vi "Dashboard Main.vi"() -> ()   [LabVIEW 2013]
uses:
  <vilib>/event_ctls.llb/eventvkey.ctl
  <vilib>/Utility/config.llb/NI_LVConfig.lvlib
  <vilib>/Utility/config.llb/Write Key (I32).vi
  <vilib>/Rock Robotics/WPI/Dashboard/WPI_DashboardLogging Global.vi
  <vilib>/Utility/config.llb/Write Key (String).vi
  2014 Robot Project/Robot Global Data.vi
panel:
  out "Image Message":string="Timeout in Camera Communications"
  in  "Rec Mode":enum32{"Stop", "Record", "Playback"}(radio)
  in  "Dashboard Tab":T1(tab)
  in  "Camera Settings":T2={"Frame Rate"=30, "Compression"=30, "Size"=1} {"Frame Rate" scale=1.0..30.0; "Size" items=["640x480", "320x240", "160x120"]}
  in  "DB Camera Config":bool
  out "fps":dbl format="%#.1g"
  out "Mbps":dbl format="%#.1g"
  out "Mbps 2":bool
  out "LED 1":bool
  in  "Slider 1":dbl(slide) scale=0.0..100.0
  in  "Checkbox 2":bool
  in  "Checkbox 1":bool
  in  "Test Slider":dbl(slide) scale=0.0..100.0 scale format="%#_3g"
  in  "On/Off":bool caption="Solenoid"
  in  "Test Name":u16(ring) items=["Select the test to run...", "Example Test", "-------------------------------", "List of tests is built in robot code.", "Replace with your own automated tests."]
  in  "Test Tree":string(tree)
  in  "Motor":cluster{"Value":dbl, "Enable":bool} {"Value" scale=-1.0..1.0 scale format="%#_3g"}
  out "Progress":T3 {"Test Progress" scale=0.0..100.0}
  in  "Rev/Fwd":cluster{"Forward":bool, "Reverse":bool}
  in  "Test Ring":u16(ring) items=["Auto", "Fixed indoor", "Fixed outdoor 1", "Fixed outdoor 2", "Fixed fluorescent 1", "Fixed fluorescent 2", "Hold current"]
  in  "Listbox":i32(listbox)
  out "Tree":string(tree)
  out "Camera Image":T4(plugin-control)
  in  "Enable":bool
  # "Left"
  # "Front"
  # "Right"
  # "Battery"
  # "Customize by placing controls and indicators here and name to\nmatch Dashboard Variables on robot."
  # "This tab is a great place for autonomous settings and validation.\nCustomize by placing controls and indicators here and name to\nmatch Dashboard Variables on robot."
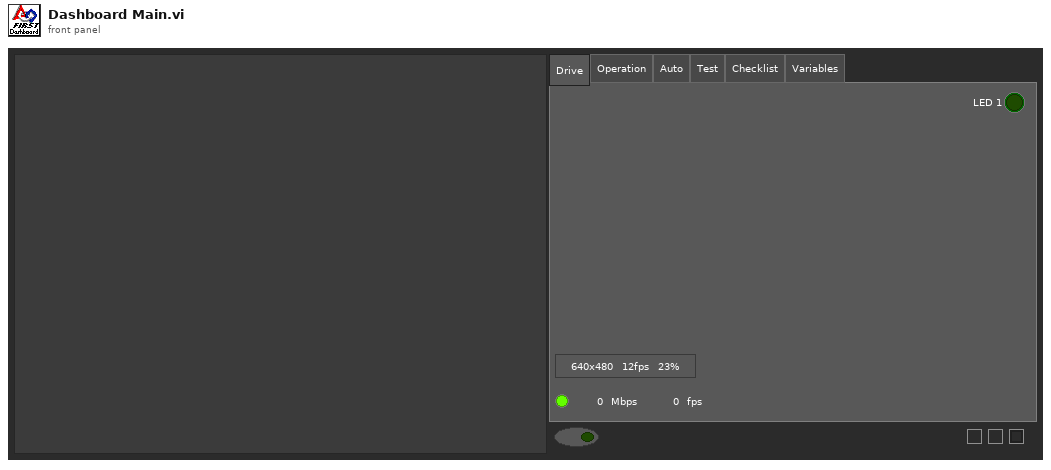
[diagram p1: front panel]
types:
  T1 = enum32{"Drive", "Operation", "Auto", "Test", "Checklist", "Variables"}
  T2 = cluster{"Frame Rate":i32, "Compression":i32, "Size":u16}
  T3 = cluster{"Test Progress":u8, "Test Progress Text":string}
  T4 = typedef "IMAQ Image.ctl" = refnum<image>
  T5 = typedef "Image Type" = u32
  T6 = typedef "NI_LVConfig.lvlib/Config Data RefNum.ctl" = refnum<k1>
  T7 = typedef "eventvkey.ctl" = enum16{"ASCII", "Enter", "Return", "Shift", "Ctrl", "Alt", "Cmd", "Opt", "Caps", "NumLock", "Clear", "Break", "Up", "Down", "Left", "Right", "Insert", "Delete", "Home", "End", "PageUp", "PageDown", "Escape", "Help", "Pause", "ScrollLock", "F1", "F2", "F3", "F4", "F5", "F6", "F7", "F8", "F9", "F10", "F11", "F12", "F13", "F14", "F15", "F16", "F17", "F18", "F19", "F20", "F21", "F22", "F23", "F24", "Play", "VolumeUp", "VolumeDown", "Mute", "Two Byte Char"}
  T8 = cluster{"Image Size":bool, "Image Type":bool, "Pixel Value":bool, "ROI Information":bool, "Zoom Factor":bool}
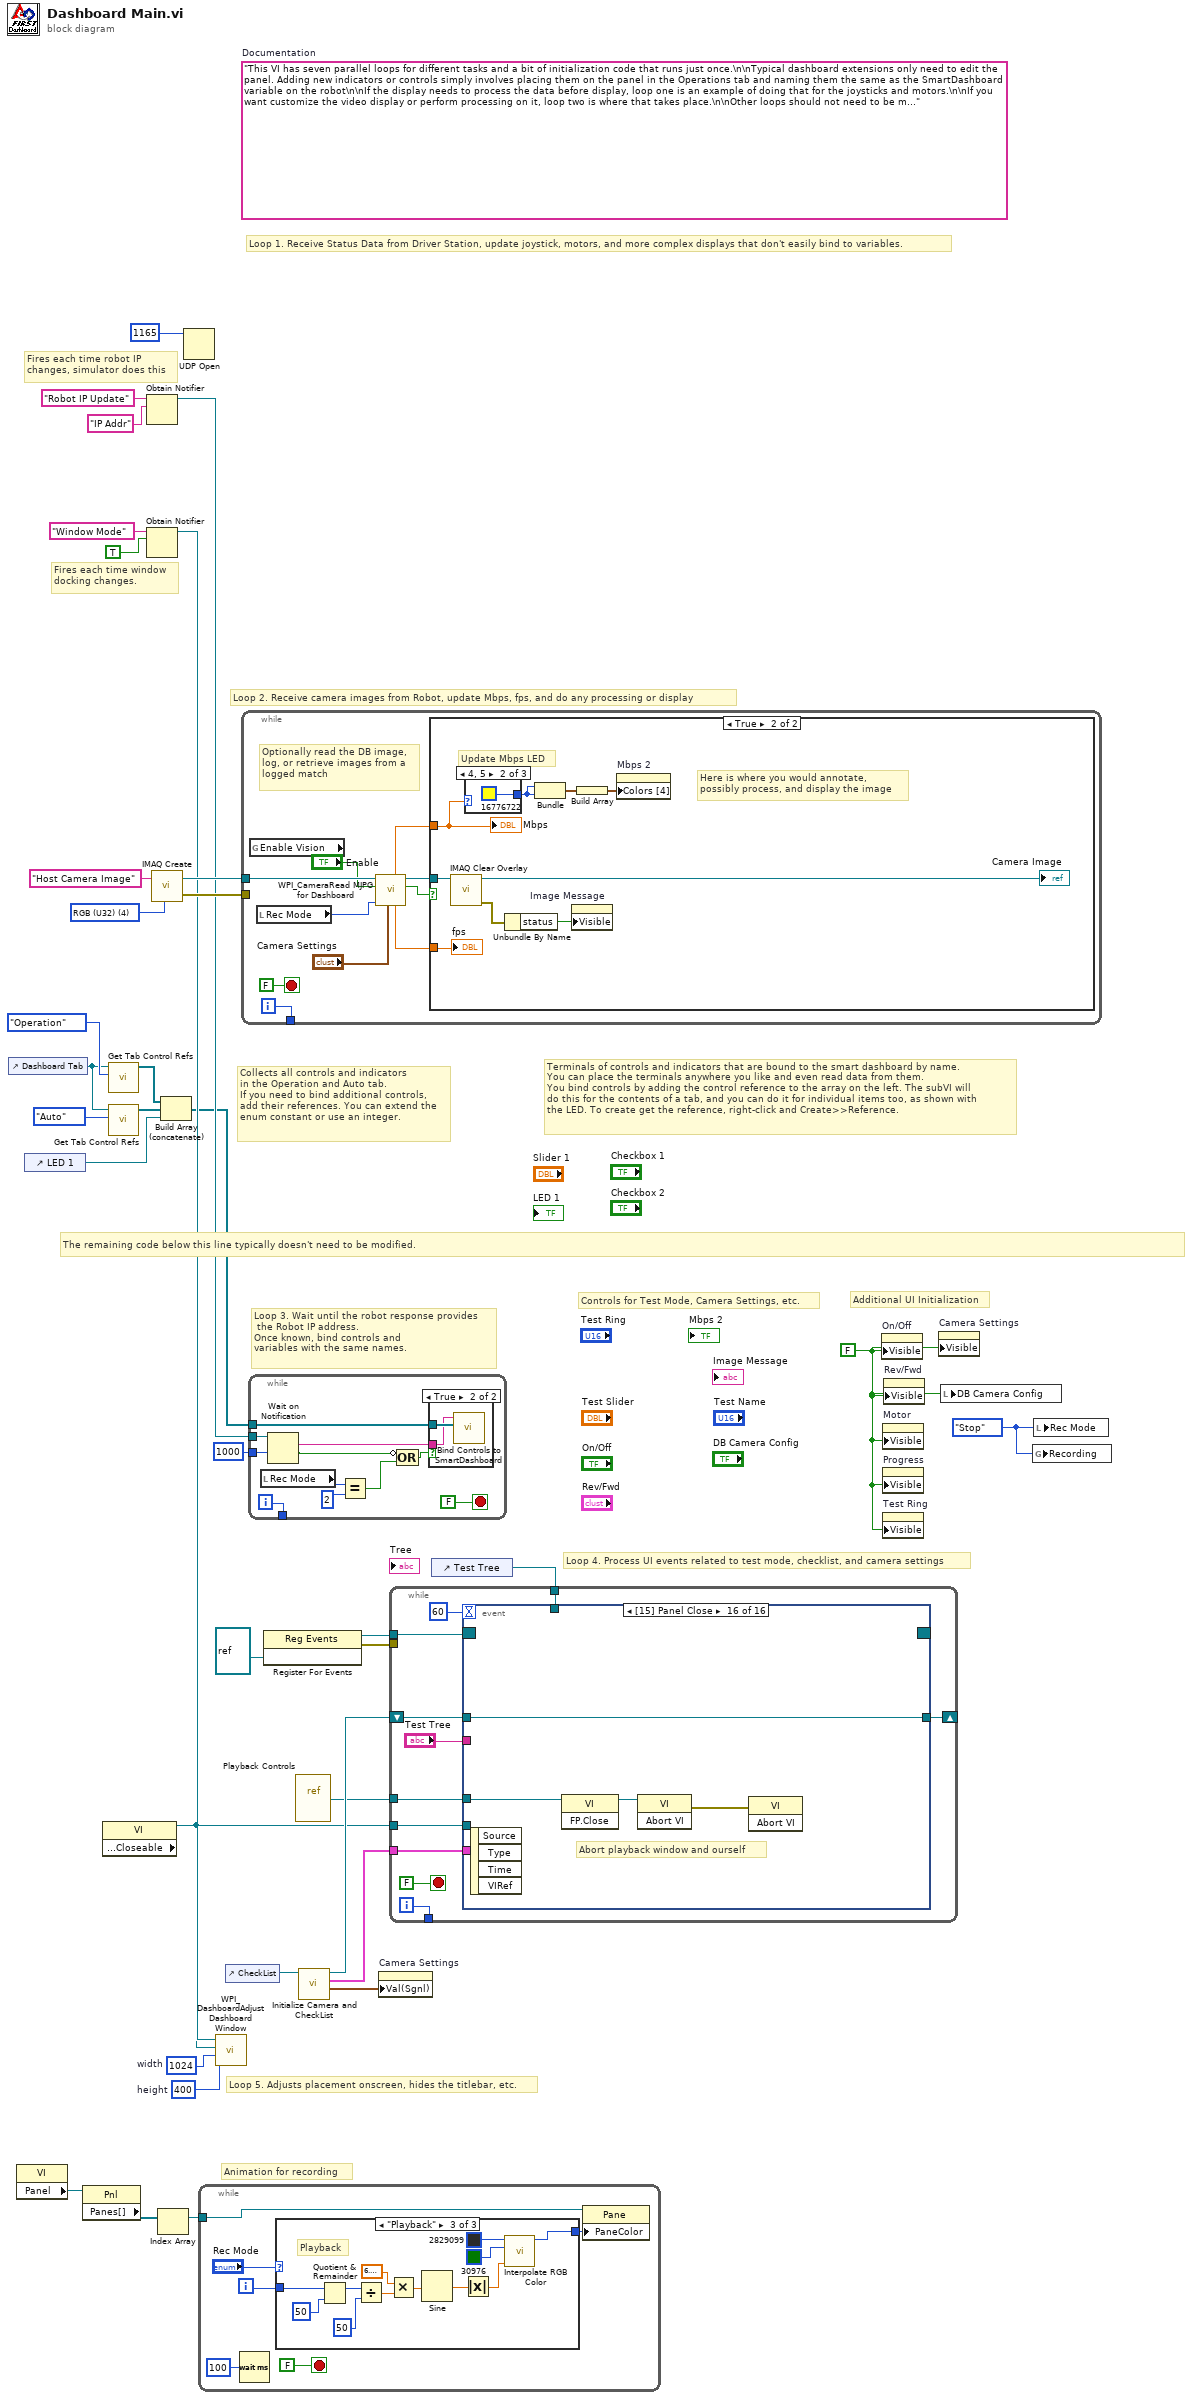
[diagram p0: block diagram]
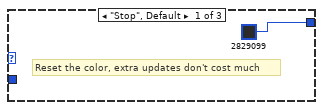
[diagram p2: hidden frame]
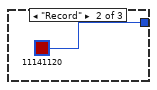
[diagram p3: hidden frame]
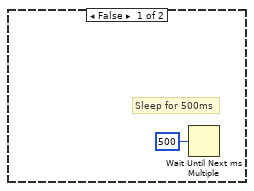
[diagram p5: hidden frame]
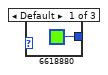
[diagram p6: hidden frame]
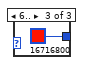
[diagram p7: hidden frame]
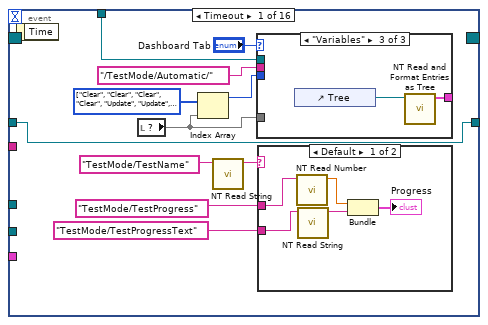
[diagram p8: hidden frame]
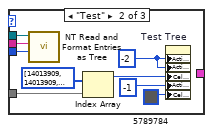
[diagram p10: hidden frame]
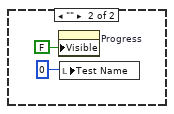
[diagram p11: hidden frame]
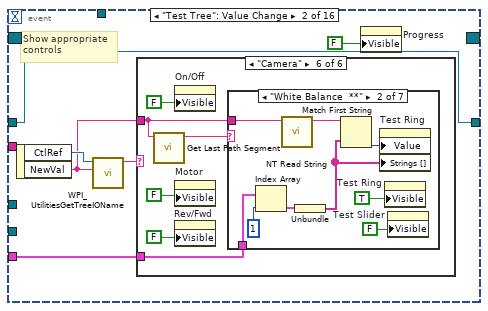
[diagram p12: hidden frame]
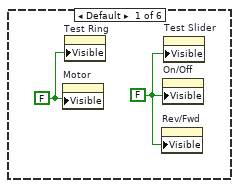
[diagram p13: hidden frame]
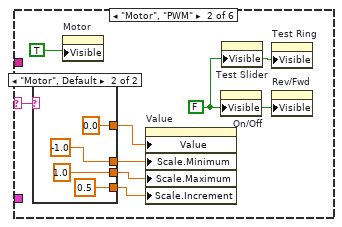
[diagram p14: hidden frame]
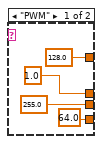
[diagram p15: hidden frame]
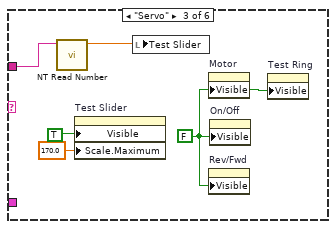
[diagram p16: hidden frame]
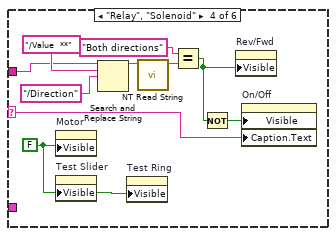
[diagram p17: hidden frame]
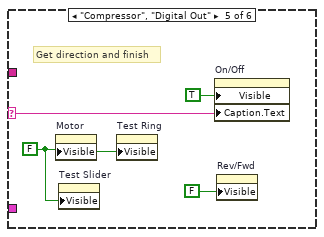
[diagram p18: hidden frame]
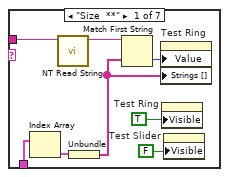
[diagram p19: hidden frame]
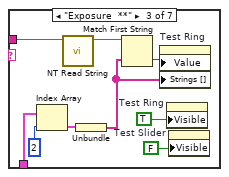
[diagram p20: hidden frame]
diagram:
  w8 = enum32{"Stop", "Record", "Playback"}."Stop" ("Rec Mode")
  w11 = 400  # height
  w12 = 1024  # width
  w25 = FALSE ("Visible")
  (unwired) "This VI has seven parallel loops for different tasks and a bit of initialization code that runs just once.\n\nTypical dashboard extensions only need to edit the panel. Adding new indicators or controls simply involves placing them on the panel in the Operations tab and naming them the same as the SmartDashboard variable on the robot\n\nIf the display needs to process the data before display, loop one is an example of doing that for the joysticks and motors.\n\nIf you want customize the video display or perform processing on it, loop two is where that takes place.\n\nOther loops should not need to be modified. They are pretty standard, and document the task they perform."  # Documentation
  w35 = T5 4 items=["Grayscale (U8)", "Grayscale (I16)", "Grayscale (SGL)", "Complex (CSG)", "RGB (U32)", "HSL (U32)", "RGB (U64)"] ("Image Type")
  # "Controls for Test Mode, Camera Settings, etc."
  # "Additional UI Initialization"
  # "Animation for recording"
  # "Fires each time robot IP\nchanges, simulator does this"
  # "Fires each time window\ndocking changes."
  # "Collects all controls and indicators\nin the Operation and Auto tab.\nIf you need to bind additional controls,\nadd their references. You can extend the\nenum constant or use an integer."
  # "The remaining code below this line typically doesn't need to be modified."
  # "Loop 4. Process UI events related to test mode, checklist, and camera settings"
  # "Terminals of controls and indicators that are bound to the smart dashboard by name.\nYou can place the terminals anywhere you like and even read data from them.\nYou bind controls by adding the control reference to the array on the left. The subVI will\ndo this for the contents of a tab, and you can do it for individual items too, as shown with\nthe LED. To create get the reference, right-click and Create>>Reference."
  # "Loop 3. Wait until the robot response provides\n the Robot IP address.\nOnce known, bind controls and\nvariables with the same names."
  # "Loop 5. Adjusts placement onscreen, hides the titlebar, etc."
  # "Loop 1. Receive Status Data from Driver Station, update joystick, motors, and more complex displays that don't easily bind to variables."
  # "Loop 2. Receive camera images from Robot, update Mbps, fps, and do any processing or display"
  n1 = control-ref of="Dashboard Tab"() -> (w6:refnum<vi>)
  n2 = property class="VI"() -> ("Panel"=w19:refnum<vi>)  [unwired: 2 in, 2 out]
  n3 = control-ref of="LED 1"() -> (w1:refnum<vi>)
  n4 = property class="Pnl"(reference=w19) -> ("Panes[]"=w20:refnum<vi>[])  [unwired: 1 in, 2 out]
  n5 = property class="VI" props=["Front Panel.Closeable"]() -> (reference out=w7:refnum<vi>)  [unwired: 2 in, 2 out]
  n6 = call <vilib>:"Get Tab Control Refs.vi"("Page Index"=T1."Operation" ("Dashboard Tab"), "TabControl in"=w6) -> ("ControlsOnPage"=w4:refnum<vi>[])  [unwired: 9 in]
  n7 = call <vilib>:"Get Tab Control Refs.vi"("Page Index"=T1."Auto" ("Dashboard Tab"), "TabControl in"=w6) -> ("ControlsOnPage"=w5:refnum<vi>[])  [unwired: 9 in]
  n8 = Obtain Notifier(name (unnamed)="Robot IP Update", notification data type="IP Addr" ("name (unnamed)")) -> (notifier out=w29:refnum<notifier>)  [unwired: 2 in, 2 out]
  n9 = Obtain Notifier(name (unnamed)="Window Mode", notification data type=TRUE) -> (notifier out=w10:refnum<notifier>)  [unwired: 2 in, 2 out]
  n10 = call "IMAQ Create"("Image Name"="Host Camera Image", "Image Type"=w35) -> ("New Image"=w33:T4, "error out"=w32:errorcluster)  [unwired: 2 in, 1 out]
  n11 = Index Array(array=w20) -> (element=w18:refnum<vi>)  [unwired: 1 in]
  n12 = Build Array (concatenate)(w4, w5, w1) -> (w3:refnum<vi>[])
  n13 = UDP Open(11:u16 1165 ("port")) -> (port=w36:refnum<k16>)  [unwired: 2 in, 4 out]
  n14 = while {
    tunnel: w18 -> [w39]
    i -> [w42]
    stop <- FALSE stop-if-true
    n15 = Wait (ms)(milliseconds to wait=u32 100) -> ()  [unwired: 1 out]
    n16 = case shown="\"Playback\"" "Rec Mode" {
      tunnel: w42 -> [_ _ w57]
      tunnel: [u32 2829099 ("Base Color") u32 11141120 ("Target Color") w46] -> w38
      frame "Stop", Default {
        # "Reset the color, extra updates don't cost much"
      }
      frame "Record" {
      }
      frame "Playback" {
        # "Playback"
        n17 = Quotient & Remainder(x=w57, y=u32 50 ("milliseconds to wait")) -> (x-y*floor(x/y)=w53:u32)  [unwired: 1 out]
        n18 = Divide(x=w53, y=u32 50 ("milliseconds to wait")) -> (x/y=w50:dbl)
        n19 = Multiply(x=6.283185307179586, y=w50) -> (x*y=w55:dbl)
        n20 = Sine(x=w55) -> (sin(x)=w54:dbl)
        n21 = Absolute Value(x=w54) -> (abs(x)=w47:dbl)
        n22 = call "Interpolate RGB Color.vi"("Proportion"=w47, "Target Color"=u32 30976, "Base Color"=u32 2829099) -> ("Result Color"=w46:u32)  [unwired: 8 in]
      }
    }
    n23 = property class="Pane"(reference=w39, "PaneColor"=w38) -> ()  [unwired: 1 in, 2 out]
  }
  n24 = call <vilib>:"WPI_DashboardAdjust Dashboard Window.vi"("height"=w11, "width"=w12, "reference in"=w7, "Notifier in"=w10) -> ()  [unwired: 8 in]
  n25 = control-ref of="CheckList"() -> (w9:refnum<vi>)
  n26 = while {
    tunnel: w33 -> [w66]
    tunnel: w32 -> [_]
    tunnel: [w67] -> _
    i -> [w67]
    stop <- FALSE stop-if-true
    # "Optionally read the DB image,\nlog, or retrieve images from a\nlogged match"
    n27 = global read "Robot Global Data.vi" "Enable Vision"() -> ()  [unwired: 1 out]
    n28 = local read "Rec Mode"() -> (w58:enum32{"Stop", "Record", "Playback"})
    n29 = call <vilib>:"WPI_CameraRead MJPG for Dashboard.vi"("Camera Settings"="Camera Settings", "Rec Mode"=w58, "Enable"="Enable", "Refnum in"=w66) -> ("Active"=w63:bool, "Refnum out"=w65:T4, "FPS"=w62:dbl, "Bandwidth (Mbps)"=w61:dbl, "Camera IP"=w59:string)  [unwired: 3 in]
    n30 = case shown="True" w63 {
      tunnel: w65 -> [_ w73]
      tunnel: w61 -> [_ w72]
      tunnel: w62 -> [_ w70]
      frame False {
        # "Sleep for 500ms"
        n31 = Wait Until Next ms Multiple(millisecond multiple=u32 500) -> ()  [unwired: 1 out]
      }
      frame True {
        # "Here is where you would annotate,\npossibly process, and display the image"
        # "Update Mbps LED"
        n32 = call "IMAQ Clear Overlay"("Image"=w73) -> ("error out"=w77:errorcluster, "Image Out"=→"Camera Image":T4)  [unwired: 2 in, 7 out]
        n33 = case shown="4, 5" w72 {
          tunnel: [u32 6618880 ("Color Box") u32 16776722 ("Color Box") u32 16716800 ("Color Box")] -> w74
          frame Default {
          }
          frame 4, 5 {
          }
          frame 6.. {
          }
        }
        n34 = Unbundle By Name(w77) -> ("status"=w78:bool)
        n35 = Bundle("Color Box"=w74, "Color Box"=w74) -> (w76:cluster{"Color Box":u32, "Color Box":u32})  [unwired: 1 out]
        n36 = property on="Image Message" class="Str"("Visible"=w78) -> ()  [unwired: 2 in, 2 out]
        n37 = Build Array(w76) -> (w75:cluster{"Color Box":u32, "Color Box":u32}[])
        n38 = property on="Mbps 2" class="Bool (strict)"("Colors [4]"=w75) -> ()  [unwired: 2 in, 2 out]
        "Mbps" <- w72
        "fps" <- w70
      }
    }
  }
  n39 = while {
    tunnel: w3 -> [w92]
    tunnel: w29 -> [w90]
    tunnel: [w88] -> _
    tunnel: u32 1000 ("milliseconds to wait") -> [w87]
    i -> [w88]
    stop <- FALSE stop-if-true
    n40 = local read "Rec Mode"() -> (w83:enum32{"Stop", "Record", "Playback"})
    n41 = Wait on Notification(notifier=w90, timeout in ms (-1)=w87) -> (notification=w89:string, timed out?=w85:bool)  [unwired: 2 in, 2 out]
    n42 = Equal?(x=w83, y=u16 2 ("Rec Mode")) -> (x = y?=w84:bool)
    n43 = Compound Arithmetic op=OR(invert w85, w84) -> (w86:bool)
    n44 = case shown="True" w86 {
      tunnel: w92 -> [_ w94]
      tunnel: w89 -> [_ w93]
      frame False {
      }
      frame True {
        n45 = call <vilib>:"Bind Controls to SmartDashboard.vi"("Bound Control Refs"=w94, "Server IP Address"=w93) -> ()  [unwired: 10 in]
      }
    }
  }
  n46 = register-events(refnum<vi> refnum) -> (reference out=w16:refnum<event-registration>, error out=w15:errorcluster)  [unwired: 2 in]
  n47 = vi-ref "Playback Controls.vi"() -> (w17:refnum<vi>)
  n48 = call "Initialize Camera and CheckList.vi"("ListBox in"=w9) -> ("Cluster"=w23:cluster{"value":i32, "value":i32, "index":i32}, "Array"=w24:cluster{string[]}[], "File Refnum"=w22:T6)  [unwired: 8 in]
  n49 = property on="Camera Settings" class="Clust (strict)"("Val(Sgnl)"=w23) -> ()  [unwired: 2 in, 2 out]
  n50 = control-ref of="Test Tree"() -> (w21:refnum<vi>)
  n51 = while {
    tunnel: w24 -> [w102]
    shift-right: [w101] -> _
    shift-left: w22 -> [w100]
    tunnel: [w99] -> _
    tunnel: w21 -> [w98]
    tunnel: w17 -> [w97]
    tunnel: w16 -> [w96]
    tunnel: w15 -> [_]
    tunnel: w7 -> [w95]
    i -> [w99]
    stop <- FALSE stop-if-true
    n52 = event shown="[15] Panel Close" {
      selector: w96 -> [_ _ _ _ _ _ _ _ _ _ _ _ _ _ _ _]
      dyn-events: [_ _ _ _ _ _ _ _ _ _ _ _ _ w340 _ _] -> _
      timeout: u32 60 ("milliseconds to wait") -> [_ _ _ _ _ _ _ _ _ _ _ _ _ _ _ _]
      tunnel: w98 -> [w112 _ _ _ _ _ _ _ _ _ _ _ _ _ _ _]
      tunnel: "Test Tree" -> [_ _ _ _ _ _ _ _ w309 w317 w319 w323 w331 _ _ _]
      tunnel: w102 -> [_ w136 _ _ _ _ w273 w303 _ _ _ _ _ _ _ _]
      tunnel: [w106 w135 w234 w239 w247 w259 w272 w296 w308 w315 w318 w322 w330 w342 w356 w357] -> w101
      tunnel: w100 -> [w106 w135 w234 w239 w247 w259 w271 w296 w308 w315 w318 w322 w330 w342 w356 w357]
      tunnel: w97 -> [_ _ _ _ _ _ _ _ _ _ _ _ _ w343 _ w360]
      tunnel: w95 -> [_ _ _ _ _ _ _ _ _ _ _ _ _ w338 _ _]
      event Timeout {
        w111 = enum16{"Update", "Clear"}[] [enum."Clear", enum."Clear", enum."Clear", enum."Clear", enum."Update", enum."Update", enum."Clear"] items=["Update", "Clear"]
        n53 = event-data() -> ()  [unwired: 1 in, 1 out]
        n54 = local read item#-1() -> (w109)
        n55 = Index Array(array=w111, index=w109) -> (element=w110:enum16{"Update", "Clear"})
        n56 = call <vilib>:"NT Read String.vi"("Name"="TestMode/TestName") -> ("String"=w115:string)  [unwired: 9 in, 1 out]
        n57 = case shown="\"Variables\"" "Dashboard Tab" {
          tunnel: w112 -> [_ w125 _]
          tunnel: "/TestMode/Automatic/" ("Name Pattern") -> [_ w124 _]
          tunnel: w110 -> [_ w123 _]
          tunnel: w109 -> [_ w121 _]
          tunnel: [_ _ w127] -> _
          frame "Operation", Default {
          }
          frame "Test" {
            w120 = -2 ("Active Item:Row Number")
            n58 = call <vilib>:"NT Read and Format Entries as Tree.vi"("Operation"=w123, "Name Pattern"=w124, "Tree Refnum"=w125) -> ()  [unwired: 7 in, 2 out]
            n59 = Index Array(array=u32[] [14013909, 14013909, 14013909, 14013909, 14013909, 16777215, 14013909], index=w121) -> (element=w119:u32)
            n60 = property on="Test Tree" class="Tree (strict)"("Active Item Row Number"=w120, "ActiveColNum"=w120, "CellBG"=w119, "Active Item Row Number"=-1 ("Active Item:Row Number"), "CellBG"=u32 5789784 ("Color Box")) -> ()  [unwired: 2 in, 2 out]
          }
          frame "Variables" {
            n61 = control-ref of="Tree"() -> (w126:refnum<vi>)
            n62 = call <vilib>:"NT Read and Format Entries as Tree.vi"("Tree Refnum"=w126) -> ("Formatted Strings"=w127:cluster{"Name":string, "Value":string}[])  [unwired: 9 in, 1 out]
          }
        }
        n63 = case shown="Default" w115 {
          tunnel: "TestMode/TestProgress" ("Name") -> [w129 _]
          tunnel: "TestMode/TestProgressText" ("Name") -> [w128 _]
          frame Default {
            n64 = call <vilib>:"NT Read Number.vi"("Name"=w129) -> ("Numeric"=w130:dbl)  [unwired: 9 in, 1 out]
            n65 = call <vilib>:"NT Read String.vi"("Name"=w128) -> ("String"=w131:string)  [unwired: 9 in, 1 out]
            n66 = Bundle("Numeric"=w130, "String"=w131) -> (→"Progress":cluster{"Numeric":dbl, "String":string})  [unwired: 1 in]
          }
          frame "" {
            n67 = property on="Progress" class="Clust (strict)"("Visible"=FALSE) -> ()  [unwired: 2 in, 2 out]
            n68 = local write "Test Name"(u16 0) -> ()
          }
        }
      }
      event "Test Tree": Value Change {
        # "Show appropriate\ncontrols"
        n69 = event-data() -> ("CtlRef"=w139:refnum<vi>, "NewVal"=w137:string)  [unwired: 1 in]
        n70 = call <vilib>:"WPI_UtilitiesGetTreeIOName.vi"("NewVal"=w137, "TreeControl in"=w139) -> ("I/O Name"=w140:string)  [unwired: 9 in]
        n71 = case shown="\"Camera\"" w140 {
          selector: w140 -> [_ w147 _ w165 w174 _]
          tunnel: w137 -> [_ _ w162 w164 _ w181]
          tunnel: w136 -> [_ _ _ _ _ w180]
          frame Default {
            w142 = FALSE ("Visible")
            w141 = FALSE ("Visible")
            n72 = property on="Motor" class="Clust (strict)"("Visible"=w141) -> ()  [unwired: 2 in, 2 out]
            n73 = property on="Test Ring" class="Ring (strict)"("Visible"=w141) -> ()  [unwired: 2 in, 2 out]
            n74 = property on="Rev/Fwd" class="Clust (strict)"("Visible"=w142) -> ()  [unwired: 2 in, 2 out]
            n75 = property on="On/Off" class="Bool (strict)"("Visible"=w142) -> ()  [unwired: 2 in, 2 out]
            n76 = property on="Test Slider" class="Slide (strict)"("Visible"=w142) -> ()  [unwired: 2 in, 2 out]
          }
          frame "Motor", "PWM" {
            w148 = FALSE ("Visible")
            n77 = case shown="\"Motor\", Default" w147 {
              tunnel: [1.0 ("Value") -1.0 ("Value")] -> w146
              tunnel: [255.0 ("Value") 1.0 ("Value")] -> w145
              tunnel: [128.0 ("Value") 0.0 ("Value")] -> w144
              tunnel: [64.0 ("Value") 0.5 ("Value")] -> w143
              frame "PWM" {
              }
              frame "Motor", Default {
              }
            }
            n78 = property on="Motor" class="Clust (strict)"("Visible"=TRUE) -> ()  [unwired: 2 in, 2 out]
            n79 = property on="Value" class="Slide (strict)"("Value"=w144, "Scale.Minimum"=w146, "Scale.Maximum"=w145, "Scale.Increment"=w143) -> ()  [unwired: 2 in, 2 out]
            n80 = property on="On/Off" class="Bool (strict)"("Visible"=w148) -> ()  [unwired: 2 in, 2 out]
            n81 = property on="Test Slider" class="Slide (strict)"("Visible"=w148) -> ()  [unwired: 2 in, 2 out]
            n82 = property on="Test Ring" class="Ring (strict)"("Visible"=w148) -> ()  [unwired: 2 in, 2 out]
            n83 = property on="Rev/Fwd" class="Clust (strict)"("Visible"=w148) -> ()  [unwired: 2 in, 2 out]
          }
          frame "Servo" {
            w160 = FALSE ("Visible")
            n84 = call <vilib>:"NT Read Number.vi"("Name"=w162) -> ("Numeric"=w161:dbl)  [unwired: 9 in, 1 out]
            n85 = property on="Test Slider" class="Slide (strict)"("Visible"=TRUE, "Scale.Maximum"=170.0 ("Scale.Range:Maximum")) -> ()  [unwired: 2 in, 2 out]
            n86 = local write "Test Slider"(w161) -> ()
            n87 = property on="Motor" class="Clust (strict)"("Visible"=w160) -> ()  [unwired: 2 in, 2 out]
            n88 = property on="Rev/Fwd" class="Clust (strict)"("Visible"=w160) -> ()  [unwired: 2 in, 2 out]
            n89 = property on="On/Off" class="Bool (strict)"("Visible"=w160) -> ()  [unwired: 2 in, 2 out]
            n90 = property on="Test Ring" class="Ring (strict)"("Visible"=w160) -> ()  [unwired: 2 in, 2 out]
          }
          frame "Relay", "Solenoid" {
            w163 = FALSE ("Visible")
            n91 = property on="Motor" class="Clust (strict)"("Visible"=w163) -> ()  [unwired: 2 in, 2 out]
            n92 = property on="Test Slider" class="Slide (strict)"("Visible"=w163) -> ()  [unwired: 2 in, 2 out]
            n93 = Search and Replace String(input string=w164, search string="/Value  **", replace string="/Direction") -> (result string=w170:string)  [unwired: 5 in, 3 out]
            n94 = property on="Test Ring" class="Ring (strict)"("Visible"=w163) -> ()  [unwired: 2 in, 2 out]
            n95 = call <vilib>:"NT Read String.vi"("Name"=w170) -> ("String"=w168:string)  [unwired: 9 in, 1 out]
            n96 = Equal?(x="Both directions", y=w168) -> (x = y?=w166:bool)
            n97 = Not(x=w166) -> (.not. x?=w167:bool)
            n98 = property on="Rev/Fwd" class="Clust (strict)"("Visible"=w166) -> ()  [unwired: 2 in, 2 out]
            n99 = property on="On/Off" class="Bool (strict)"("Visible"=w167, "Caption.Text"=w165) -> ()  [unwired: 2 in, 2 out]
          }
          frame "Compressor", "Digital Out" {
            w173 = FALSE ("Visible")
            # "Get direction and finish"
            n100 = property on="Motor" class="Clust (strict)"("Visible"=w173) -> ()  [unwired: 2 in, 2 out]
            n101 = property on="Test Slider" class="Slide (strict)"("Visible"=w173) -> ()  [unwired: 2 in, 2 out]
            n102 = property on="Test Ring" class="Ring (strict)"("Visible"=w173) -> ()  [unwired: 2 in, 2 out]
            n103 = property on="On/Off" class="Bool (strict)"("Visible"=TRUE, "Caption.Text"=w174) -> ()  [unwired: 2 in, 2 out]
            n104 = property on="Rev/Fwd" class="Clust (strict)"("Visible"=FALSE) -> ()  [unwired: 2 in, 2 out]
          }
          frame "Camera" {
            n105 = call <vilib>:"Get Last Path Segment.vi"("String in"=w181) -> ("String out"=w182:string)  [unwired: 10 in]
            n106 = property on="On/Off" class="Bool (strict)"("Visible"=FALSE) -> ()  [unwired: 2 in, 2 out]
            n107 = property on="Motor" class="Clust (strict)"("Visible"=FALSE) -> ()  [unwired: 2 in, 2 out]
            n108 = property on="Rev/Fwd" class="Clust (strict)"("Visible"=FALSE) -> ()  [unwired: 2 in, 2 out]
            n109 = case shown="\"White Balance  **\"" w182 {
              tunnel: w181 -> [w188 w197 w206 w215 w224 _ w230]
              tunnel: w180 -> [w186 w194 w203 w212 w221 _ _]
              frame "Size  **" {
                n110 = Index Array(array=w186) -> (element=w185:cluster{string[]})  [unwired: 1 in]
                n111 = call <vilib>:"NT Read String.vi"("Name"=w188) -> ("String"=w187:string)  [unwired: 9 in, 1 out]
                n112 = Unbundle(w185) -> (w183:string[])
                n113 = Match First String(2:w183, 3:w187) -> (0:w184:i32)  [unwired: 1 out]
                n114 = property on="Test Ring" class="Ring (strict)"("Value"=w184, "Strings []"=w183) -> ()  [unwired: 2 in, 2 out]
                n115 = property on="Test Ring" class="Ring (strict)"("Visible"=TRUE) -> ()  [unwired: 2 in, 2 out]
                n116 = property on="Test Slider" class="Slide (strict)"("Visible"=FALSE) -> ()  [unwired: 2 in, 2 out]
              }
              frame "White Balance  **" {
                n117 = Index Array(array=w194, index=1) -> (element=w195:cluster{string[]})
                n118 = call <vilib>:"NT Read String.vi"("Name"=w197) -> ("String"=w196:string)  [unwired: 9 in, 1 out]
                n119 = Unbundle(w195) -> (w192:string[])
                n120 = Match First String(2:w192, 3:w196) -> (0:w191:i32)  [unwired: 1 out]
                n121 = property on="Test Ring" class="Ring (strict)"("Value"=w191, "Strings []"=w192) -> ()  [unwired: 2 in, 2 out]
                n122 = property on="Test Ring" class="Ring (strict)"("Visible"=TRUE) -> ()  [unwired: 2 in, 2 out]
                n123 = property on="Test Slider" class="Slide (strict)"("Visible"=FALSE) -> ()  [unwired: 2 in, 2 out]
              }
              frame "Exposure  **" {
                n124 = Index Array(array=w203, index=2) -> (element=w204:cluster{string[]})
                n125 = call <vilib>:"NT Read String.vi"("Name"=w206) -> ("String"=w205:string)  [unwired: 9 in, 1 out]
                n126 = Unbundle(w204) -> (w200:string[])
                n127 = Match First String(2:w200, 3:w205) -> (0:w201:i32)  [unwired: 1 out]
                n128 = property on="Test Ring" class="Ring (strict)"("Value"=w201, "Strings []"=w200) -> ()  [unwired: 2 in, 2 out]
                n129 = property on="Test Ring" class="Ring (strict)"("Visible"=TRUE) -> ()  [unwired: 2 in, 2 out]
                n130 = property on="Test Slider" class="Slide (strict)"("Visible"=FALSE) -> ()  [unwired: 2 in, 2 out]
              }
              frame "Exposure Priority  **" {
                n131 = Index Array(array=w212, index=3) -> (element=w213:cluster{string[]})
                n132 = call <vilib>:"NT Read String.vi"("Name"=w215) -> ("String"=w214:string)  [unwired: 9 in, 1 out]
                n133 = Unbundle(w213) -> (w209:string[])
                n134 = Match First String(2:w209, 3:w214) -> (0:w210:i32)  [unwired: 1 out]
                n135 = property on="Test Ring" class="Ring (strict)"("Value"=w210, "Strings []"=w209) -> ()  [unwired: 2 in, 2 out]
                n136 = property on="Test Ring" class="Ring (strict)"("Visible"=TRUE) -> ()  [unwired: 2 in, 2 out]
                n137 = property on="Test Slider" class="Slide (strict)"("Visible"=FALSE) -> ()  [unwired: 2 in, 2 out]
              }
              frame "Color Enable  **" {
                n138 = Index Array(array=w221, index=4) -> (element=w222:cluster{string[]})
                n139 = call <vilib>:"NT Read String.vi"("Name"=w224) -> ("String"=w223:string)  [unwired: 9 in, 1 out]
                n140 = Unbundle(w222) -> (w218:string[])
                n141 = Match First String(2:w218, 3:w223) -> (0:w219:i32)  [unwired: 1 out]
                n142 = property on="Test Ring" class="Ring (strict)"("Value"=w219, "Strings []"=w218) -> ()  [unwired: 2 in, 2 out]
                n143 = property on="Test Ring" class="Ring (strict)"("Visible"=TRUE) -> ()  [unwired: 2 in, 2 out]
                n144 = property on="Test Slider" class="Slide (strict)"("Visible"=FALSE) -> ()  [unwired: 2 in, 2 out]
              }
              frame Default {
                n145 = property on="Test Ring" class="Ring (strict)"("Visible"=FALSE) -> ()  [unwired: 2 in, 2 out]
                n146 = property on="Test Slider" class="Slide (strict)"("Visible"=FALSE) -> ()  [unwired: 2 in, 2 out]
              }
              frame "Brightness  **", "Color Level  **", "Compression  **", "FPS  **", "Sharpness  **" {
                n147 = call <vilib>:"NT Read Number.vi"("Name"=w230) -> ("Numeric"=w229:dbl)  [unwired: 9 in, 1 out]
                n148 = local write "Test Slider"(w229) -> ()
                n149 = property on="Test Slider" class="Slide (strict)"("Visible"=TRUE, "Scale.Maximum"=100.0 ("Scale.Range:Maximum")) -> ()  [unwired: 2 in, 2 out]
                n150 = property on="Test Ring" class="Ring (strict)"("Visible"=FALSE) -> ()  [unwired: 2 in, 2 out]
              }
            }
          }
        }
        n151 = property on="Progress" class="Clust (strict)"("Visible"=FALSE) -> ()  [unwired: 2 in, 2 out]
      }
      event "Test Name": Mouse Enter {
        # "Populate the ring with the list of tests"
        n152 = event-data() -> ()  [unwired: 1 in, 1 out]
        n153 = call <vilib>:"NT Read String Array.vi"("Name"="TestMode/TestList") -> ("String Array"=w238:string[])  [unwired: 9 in, 1 out]
        n154 = Build Array (concatenate)("Select the test to run...", w238) -> (w237:string[])
        n155 = property on="Test Name" class="Ring (strict)"("Strings []"=w237) -> ()  [unwired: 2 in, 2 out]
      }
      event "Test Name": Value Change {
        w240 = FALSE ("Visible")
        # "Tell the robot the test name to run"
        n156 = event-data() -> ("NewVal"=w244:u16)  [unwired: 1 in]
        n157 = property on="Test Name" class="Ring (strict)"() -> ("Strings []"=w245:string[])  [unwired: 2 in, 2 out]
        n158 = local write "Progress"(T3 {"Test Progress"=0, "Test Progress Text"=""} ("Progress")) -> ()
        n159 = Index Array(array=w245, index=w244) -> (element=w243:string)
        n160 = call <vilib>:"NT Write String.vi"("String"=w243, "Name"="TestMode/TestName") -> ()  [unwired: 9 in, 1 out]
        n161 = property on="Progress" class="Clust (strict)"("Visible"=TRUE) -> ()  [unwired: 2 in, 2 out]
        n162 = property on="Motor" class="Clust (strict)"("Visible"=w240) -> ()  [unwired: 2 in, 2 out]
        n163 = property on="Test Slider" class="Slide (strict)"("Visible"=w240) -> ()  [unwired: 2 in, 2 out]
        n164 = property on="On/Off" class="Bool (strict)"("Visible"=w240) -> ()  [unwired: 2 in, 2 out]
        n165 = property on="Rev/Fwd" class="Clust (strict)"("Visible"=w240) -> ()  [unwired: 2 in, 2 out]
        n166 = property on="Test Ring" class="Ring (strict)"("Visible"=w240) -> ()  [unwired: 2 in, 2 out]
      }
      event "Listbox": Double Click {
        n167 = event-data() -> ("PlatMods.Shift"=w248:bool, "Row"=w250:i32)  [unwired: 1 in]
        n168 = case shown="True" w248 {
          tunnel: w250 -> [w254 _]
          tunnel: 1 -> [w253 _]
          frame False {
            n169 = property on="Listbox" class="LstBox (strict)"() -> ("Item Symbols"=w252:i32[])  [unwired: 2 in, 2 out]
            n170 = Replace Array Subset(array=w252, new element=w253, index=w254) -> (w251:i32[])
            n171 = property on="Listbox" class="LstBox (strict)"("Item Symbols"=w251) -> ()  [unwired: 2 in, 2 out]
          }
          frame True {
            w255 = 0 ("Top Row")
            n172 = property on="Listbox" class="LstBox (strict)"() -> ("Number of Rows"=w257:u32)  [unwired: 2 in, 2 out]
            n173 = Initialize Array(0, w257) -> (w256:i32[])
            n174 = property on="Listbox" class="LstBox (strict)"("Top Row"=w255, "Value"=w255, "Item Symbols"=w256) -> ()  [unwired: 2 in, 2 out]
          }
        }
      }
      event "Listbox": Key Down {
        n175 = event-data() -> ("VKey"=w261:T7)  [unwired: 1 in]
        n176 = case shown="\"Left\", \"Right\"" w261 {
          selector: w261 -> [w266 _]
          tunnel: eventvkey."Left" ("VKey") -> [w264 _]
          frame "Left", "Right" {
            n177 = Equal?(x=w264, y=w266) -> (x = y?=w265:bool)
            n178 = Select(t=0, s=w265, f=1) -> (s? t:f=w267:i32)
            n179 = property on="Listbox" class="LstBox (strict)"() -> ("Item Symbols"=w270:i32[])  [unwired: 2 in, 2 out]
            n180 = Replace Array Subset(array=w270, new element=w267, index="Listbox") -> (w269:i32[])
            n181 = property on="Listbox" class="LstBox (strict)"("Item Symbols"=w269) -> ()  [unwired: 2 in, 2 out]
          }
          frame Default {
          }
        }
      }
      event "DB Camera Config": Value Change {
        n182 = event-data() -> ("NewVal"=w274:bool)  [unwired: 1 in]
        n183 = case shown="False" w274 {
          tunnel: w273 -> [w283 _]
          tunnel: [w276 w294] -> w272
          tunnel: w271 -> [w275 w294]
          frame False {
            w290 = "Camera"
            w293 = FALSE ("Visible")
            n184 = local read "Camera Settings"() -> (w282:T2)
            n185 = Index Array(array=w283) -> (element=w286:cluster{string[]})  [unwired: 1 in]
            n186 = Unbundle(w282) -> ("Frame Rate"=w281:i32, "Compression"=w280:i32, "Size"=w284:u16)
            n187 = Unbundle(w286) -> (w285:string[])
            n188 = Index Array(array=w285, index=w284) -> (element=w279:string)
            n189 = call-poly <vilib>:"Write Key.vi"("section"=w290, "value"=w279, "key"="Size", "refnum"=w275) -> ("refnum out"=w292:T6)  [unwired: 2 in, 5 out]
            n190 = call-poly <vilib>:"Write Key.vi"("section"=w290, "value"=w281, "key"="FrameRate", "refnum"=w292) -> ("refnum out"=w291:T6)  [unwired: 1 in, 6 out]
            n191 = property on="Camera Settings" class="Clust (strict)"("Visible"=w293) -> ()  [unwired: 2 in, 2 out]
            n192 = local write "DB Camera Config"(w293) -> ()
            n193 = call-poly <vilib>:"Write Key.vi"("section"=w290, "value"=w280, "key"="Compression", "refnum"=w291) -> ("refnum out"=w277:T6)  [unwired: 1 in, 6 out]
            n194 = call <vilib>:"Close Config Data.vi"("refnum"=w277) -> ("file path"=w278:path)  [unwired: 2 in, 8 out]
            n195 = call <vilib>:"Open Config Data.vi"("configuration file path"=w278) -> ("refnum"=w276:T6)  [unwired: 8 in, 2 out]
          }
          frame True {
            n196 = property on="Camera Settings" class="Clust (strict)"("Visible"=TRUE) -> ()  [unwired: 2 in, 2 out]
          }
        }
      }
      event "Camera Settings": Value Change {
        n197 = event-data() -> ("NewVal"=w307:T2)  [unwired: 1 in]
        n198 = Index Array(array=w303) -> (element=w302:cluster{string[]})  [unwired: 1 in]
        n199 = Unbundle(w307) -> ("Frame Rate"=w298:i32, "Compression"=w297:i32, "Size"=w300:u16)
        n200 = Unbundle(w302) -> (w301:string[])
        n201 = Index Array(array=w301, index=w300) -> (element=w299:string)
        n202 = Format Into String(format string="%s   %dfps   %d%%", w299, w298, w297) -> (resulting string=w304:string)  [unwired: 2 in, 1 out]
        n203 = Build Array(w304) -> (w305:string[])
        n204 = property on="DB Camera Config" class="Bool (strict)"("Strings [4]"=w305) -> ()  [unwired: 2 in, 2 out]
      }
      event "Motor.Enable": Value Change {
        n205 = event-data() -> ("NewVal"=w313:bool)  [unwired: 1 in]
        n206 = Unbundle("Motor") -> ("Value"=w312:dbl)  [unwired: 1 out]
        n207 = Select(t=w312, s=w313, f=0.0) -> (s? t:f=w310:dbl)
        n208 = call <vilib>:"NT Write Number.vi"("Numeric"=w310, "Name"=w309) -> ()  [unwired: 9 in, 1 out]
      }
      event "Test Slider": Value Change {
        n209 = event-data() -> ("NewVal"=w316:dbl)  [unwired: 1 in]
        n210 = call <vilib>:"NT Write Number.vi"("Numeric"=w316, "Name"=w317) -> ()  [unwired: 9 in, 1 out]
      }
      event "On/Off": Value Change {
        n211 = event-data() -> ("NewVal"=w321:bool)  [unwired: 1 in]
        n212 = Boolean To (0,1)(Boolean=w321) -> (0, 1=w320:i16)
        n213 = call <vilib>:"NT Write Number.vi"("Numeric"=w320, "Name"=w319) -> ()  [unwired: 9 in, 1 out]
      }
      event "Rev/Fwd": Value Change {
        n214 = event-data() -> ("NewVal.Forward"=w329:bool, "NewVal.Reverse"=w328:bool)  [unwired: 1 in]
        n215 = Boolean To (0,1)(Boolean=w329) -> (0, 1=w325:i16)
        n216 = Boolean To (0,1)(Boolean=w328) -> (0, 1=w327:i16)
        n217 = Negate(x=w327) -> (-x=w326:i16)
        n218 = Add(x=w325, y=w326) -> (x+y=w324:i16)
        n219 = call <vilib>:"NT Write Number.vi"("Numeric"=w324, "Name"=w323) -> ()  [unwired: 9 in, 1 out]
      }
      event "Test Ring": Value Change {
        n220 = event-data() -> ("NewVal"=w333:u16)  [unwired: 1 in]
        n221 = property on="Test Ring" class="Ring (strict)"() -> ("Strings []"=w334:string[])  [unwired: 2 in, 2 out]
        n222 = Index Array(array=w334, index=w333) -> (element=w332:string)
        n223 = call <vilib>:"NT Write String.vi"("String"=w332, "Name"=w331) -> ()  [unwired: 9 in, 1 out]
      }
      event "Rec Mode": Value Change {
        # "Update globals for recording mode and path to read log from.\nClear when logging and let NetworkTables set path for vision to\nuse."
        n224 = event-data() -> ("NewVal"=w344:enum32{"Stop", "Record", "Playback"})  [unwired: 1 in]
        n225 = global write "WPI_DashboardLogging Global.vi" "Logging Filename"(path "") -> ()
        n226 = case shown="\"Stop\", \"Record\"" w344 {
          tunnel: w343 -> [_ w346 w354]
          tunnel: [_ _ w353] -> w340
          tunnel: [_ _ w352] -> _
          tunnel: w338 -> [_ _ w350]
          tunnel: cluster{i32, i32} {-250, 170} -> [_ _ w349]
          tunnel: [_ _ T8 {"Image Size"=TRUE, "Image Type"=TRUE, "Pixel Value"=TRUE, "ROI Information"=TRUE, "Zoom Factor"=FALSE} ("Image Information Shown:All Elements")] -> w336
          tunnel: [_ _ TRUE ("Zoom Factor")] -> w335
          frame Default {
          }
          frame "Stop", "Record" {
            # "Place Window too"
            n227 = invoke class="VI" method="FP.Close"(reference=w346) -> (reference out=w345:refnum<vi>)  [unwired: 2 in, 2 out]
            n228 = invoke class="VI" method="Abort VI"(reference=w345) -> ()  [unwired: 2 in, 3 out]
          }
          frame "Playback" {
            n229 = call "Open Playback Panel.vi"("Offset"=w349, "DB VI Ref"=w350, "Playback in"=w354) -> ("Playback out"=w351:refnum<vi>)  [unwired: 8 in]
            n230 = register-events(w351) -> (reference out=w353:refnum<event-registration>, error out=w352:errorcluster)  [unwired: 2 in]
          }
        }
        n231 = global write "WPI_DashboardLogging Global.vi" "Recording"(w344) -> ()
        n232 = property on="Camera Image" class="ImageControl"("Image Information Shown"=w336, "Image Information Visible"=w335) -> ()  [unwired: 2 in, 2 out]
        n233 = call <vilib>:"WPI_DashboardNT Log FieldName Cache.vi"("Operation"=enum16{"Lookup/Add", "Index", "Clear"}."Clear") -> ()  [unwired: 8 in, 3 out]
      }
      event Panel Close {
        w355 = enum32{"Stop", "Record", "Playback"}."Stop" ("Rec Mode")
        n234 = event-data() -> ()  [unwired: 1 in, 4 out]
        n235 = local write "Rec Mode"(w355) -> ()
        n236 = global write "WPI_DashboardLogging Global.vi" "Recording"(w355) -> ()
      }
      event Panel Close {
        # "Abort playback window and ourself"
        n237 = event-data() -> ()  [unwired: 1 in, 4 out]
        n238 = invoke class="VI" method="FP.Close"(reference=w360) -> (reference out=w359:refnum<vi>)  [unwired: 2 in, 2 out]
        n239 = invoke class="VI" method="Abort VI"(reference=w359) -> (error out=w358:errorcluster)  [unwired: 2 in, 2 out]
        n240 = invoke class="VI" method="Abort VI"(error in=w358) -> ()  [unwired: 2 in, 3 out]
      }
    }
  }
  n241 = property on="On/Off" class="Bool (strict)"("Visible"=w25) -> ()  [unwired: 2 in, 2 out]
  n242 = property on="Motor" class="Clust (strict)"("Visible"=w25) -> ()  [unwired: 2 in, 2 out]
  n243 = property on="Progress" class="Clust (strict)"("Visible"=w25) -> ()  [unwired: 2 in, 2 out]
  n244 = property on="Test Ring" class="Ring (strict)"("Visible"=w25) -> ()  [unwired: 2 in, 2 out]
  n245 = property on="Rev/Fwd" class="Clust (strict)"("Visible"=w25) -> ()  [unwired: 2 in, 2 out]
  n246 = property on="Camera Settings" class="Clust (strict)"("Visible"=w25) -> ()  [unwired: 2 in, 2 out]
  n247 = local write "DB Camera Config"(w25) -> ()
  n248 = global write "WPI_DashboardLogging Global.vi" "Recording"(w8) -> ()
  n249 = local write "Rec Mode"(w8) -> ()
